vi "Coffee_Main.vi"() -> ()   [LabVIEW 2020]
doc: "This VI performs the application of coffee machine controller where user can choose the beverage."
uses:
  Controls/QueueOperations.ctl
  Controls/DataCluster.ctl
  <vilib>/Utility/config.llb/Read Key (Boolean).vi
  <vilib>/Utility/config.llb/Read Key (I32).vi
  <vilib>/Utility/config.llb/Read Key (Double).vi
  <vilib>/Utility/config.llb/NI_LVConfig.lvlib
panel:
  in  "Power":bool
  out "error out":errorcluster
  in  "error in (no error)":errorcluster
  in  "Dispenser":dbl(slide) scale=0.0..60.0
  in  "Chamber":dbl(slide) scale=0.0..60.0
  out "Milk level":dbl(slide) scale=0.0..100.0
  out "Water Level":dbl(slide) scale=0.0..100.0
  out "Bean Level":dbl(slide) scale=0.0..100.0
  out "Total Cups":i32
  out "Elapsed Time":dbl
  out "Dispensing":bool
  out "Brewing":bool
  out "Grinding":bool
  out "Purging":bool
  out "Heating":bool
  out "Low Milk":bool
  out "Low Bean":bool
  out "Low Water":bool
  in  "1 Carale":bool
  in  "1 Cup":bool
  in  "Knob":i32(knob) scale=0.0..2.0
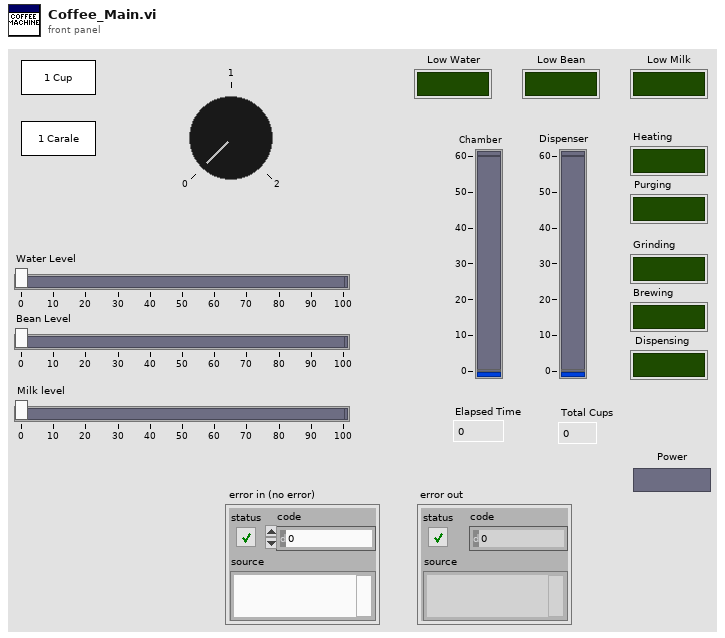
[diagram p1: front panel]
types:
  T1 = typedef "DataCluster.ctl" = cluster{"Brewing":bool, "Grinding":bool, "Purging":bool, "Dispensing":bool, "Heating":bool, "Low Milk":bool, "Low Bean":bool, "Low Water":bool, "Path":path, "Power On?":bool, "Proper Shutdown?":bool, "Total Cups":i32, "Start Time":dbl, "Elapsed Time":dbl, "Bean Level":dbl, "Milk Level":dbl, "Water Level":dbl, "HeatTime":dbl, "Beverage Type":string, "Steps":string[], "Time Sequence":dbl[], "Index":i32}
  T2 = typedef "QueueOperations.ctl" = enum16{"Create", "Enqueue", "Enqueue N", "Enstack", "Dequeue", "Flush", "Release"}
  T3 = typedef "NI_LVConfig.lvlib/Config Data RefNum.ctl" = refnum<k1>
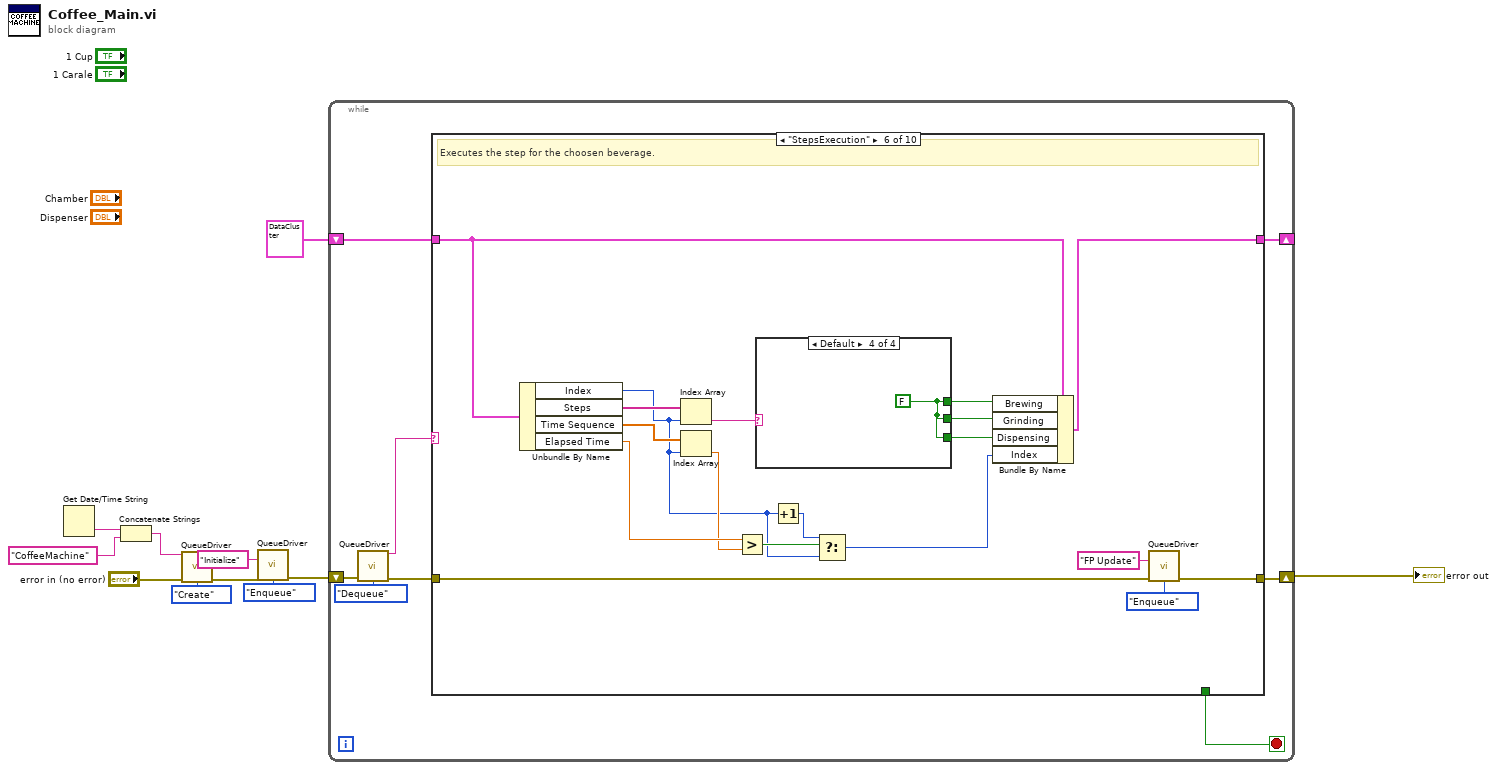
[diagram p0: block diagram]
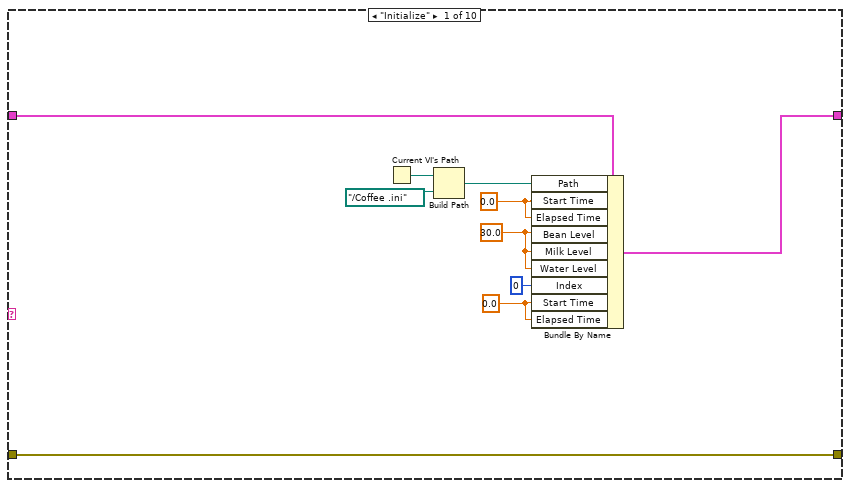
[diagram p2: hidden frame]
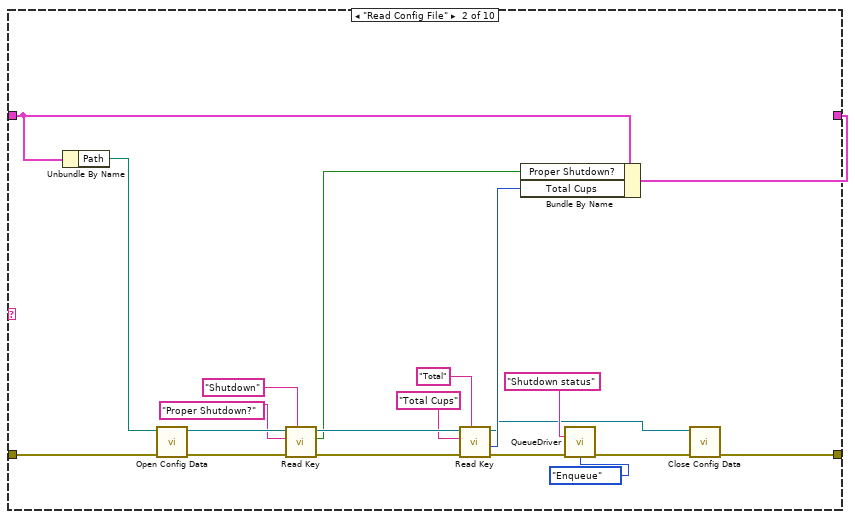
[diagram p3: hidden frame]
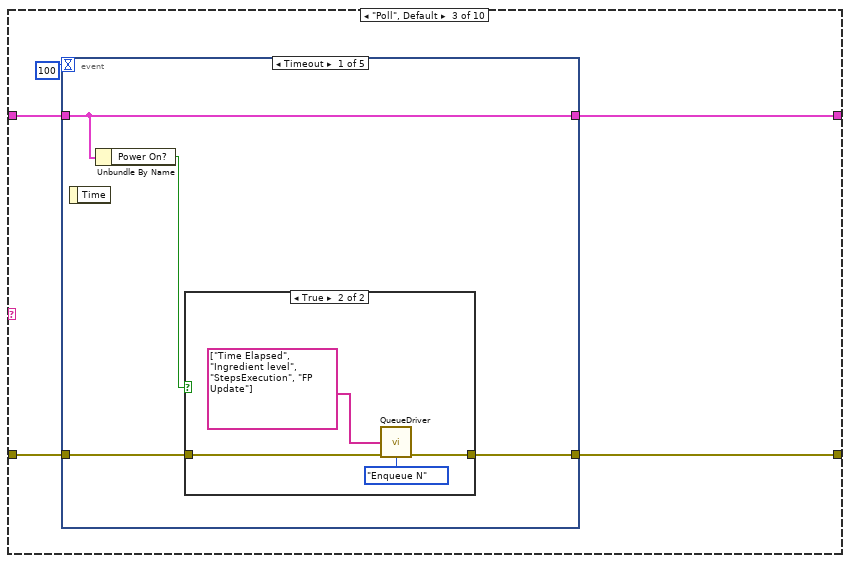
[diagram p4: hidden frame]
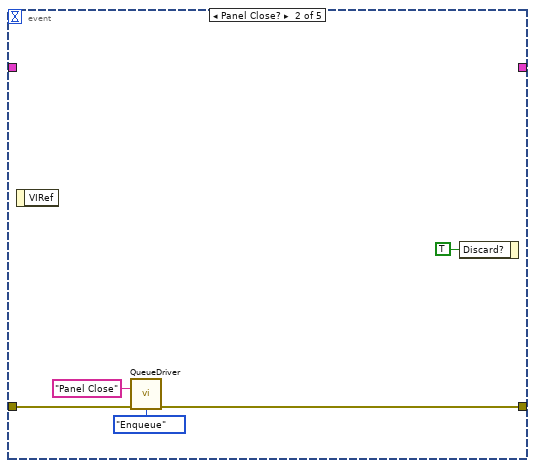
[diagram p6: hidden frame]
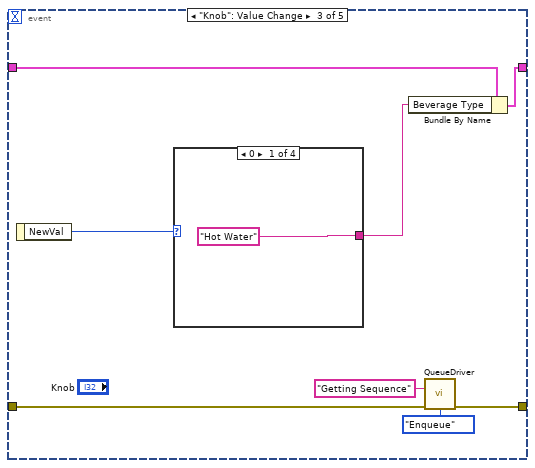
[diagram p7: hidden frame]
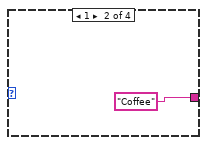
[diagram p8: hidden frame]
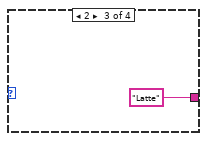
[diagram p9: hidden frame]
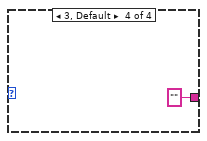
[diagram p10: hidden frame]
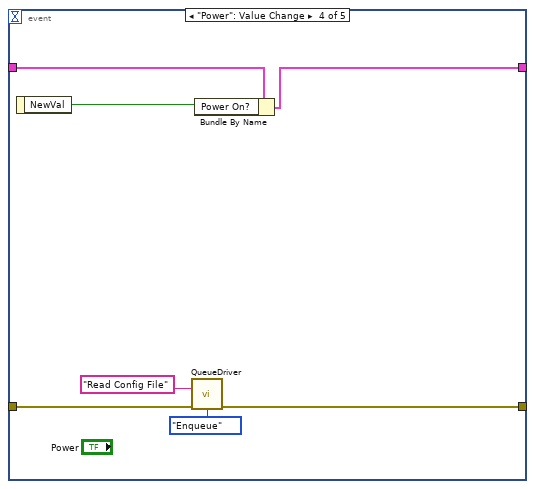
[diagram p11: hidden frame]
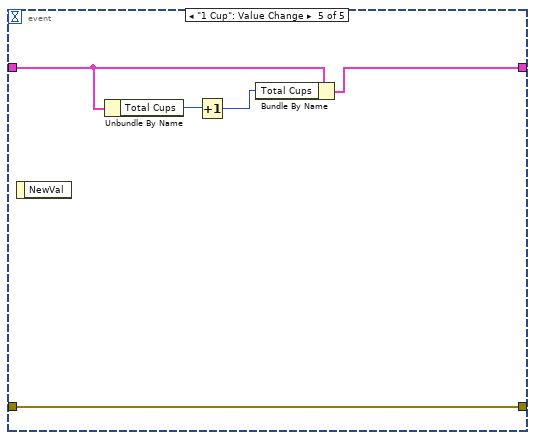
[diagram p12: hidden frame]
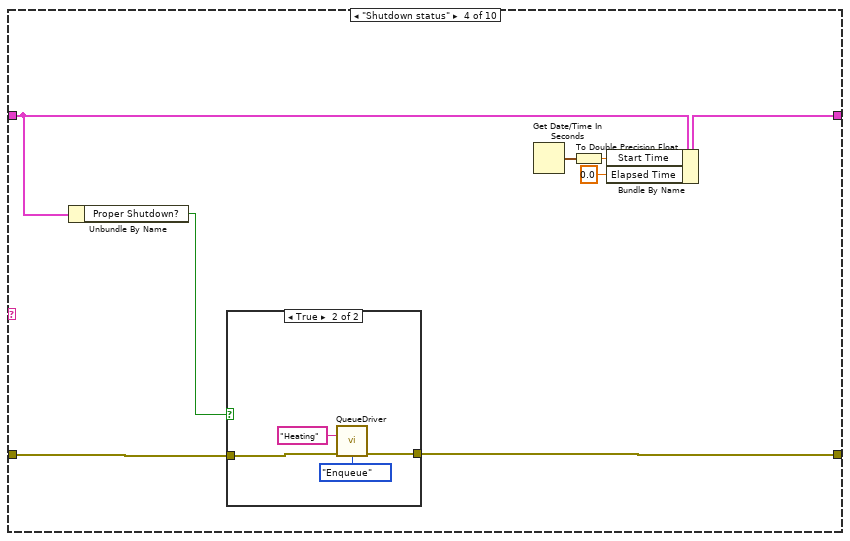
[diagram p13: hidden frame]
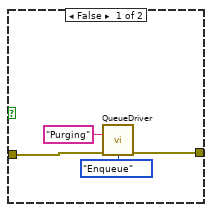
[diagram p14: hidden frame]
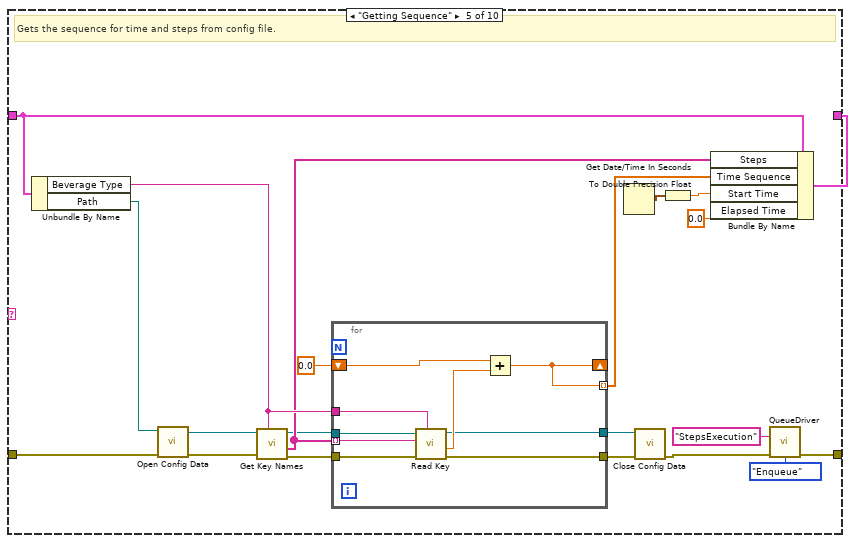
[diagram p15: hidden frame]
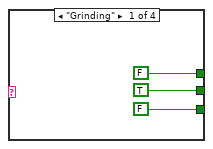
[diagram p16: hidden frame]
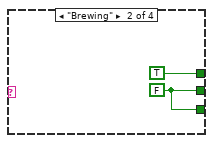
[diagram p17: hidden frame]
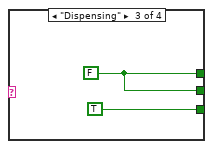
[diagram p18: hidden frame]
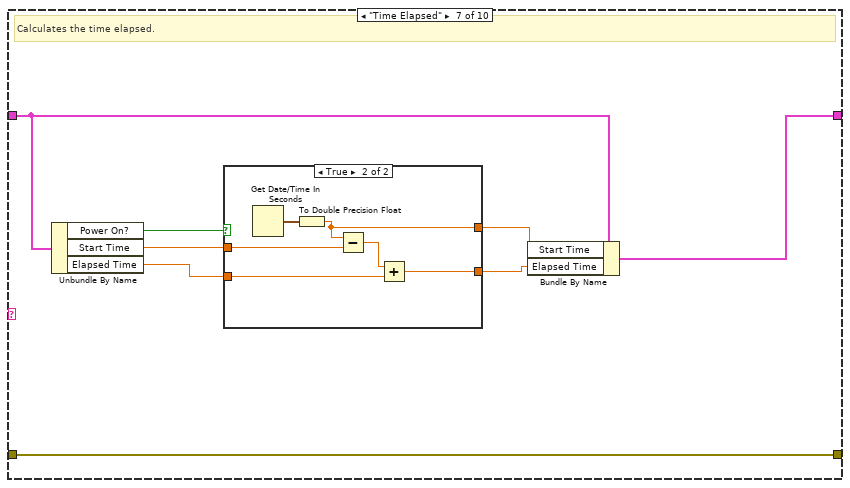
[diagram p19: hidden frame]
diagram:
  n1 = Get Date/Time String() -> (time string=w9:string)  [unwired: 3 in, 1 out]
  n2 = Concatenate Strings(w9, "CoffeeMachine" ("Queue Name")) -> (w10:string)
  n3 = call "QueueDriver.vi"("Queue Name"=w10, "error in (no error)"="error in (no error)", "Operation"=QueueOperations."Create") -> ("error out"=w6:errorcluster)  [unwired: 11 in, 1 out]
  n4 = call "QueueDriver.vi"("State"="Initialize", "error in (no error)"=w6, "Operation"=QueueOperations."Enqueue") -> ("error out"=w4:errorcluster)  [unwired: 11 in, 1 out]
  n5 = while {
    shift-right: [w14] -> _
    shift-left: T1 {"Brewing"=FALSE, "Grinding"=FALSE, "Purging"=FALSE, "Dispensing"=FALSE, "Heating"=FALSE, "Low Milk"=FALSE, "Low Bean"=FALSE, "Low Water"=FALSE, "Path"=path "", "Power On?"=FALSE, "Proper Shutdown?"=FALSE, "Total Cups"=0, "Start Time"=0.0, "Elapsed Time"=0.0, "Bean Level"=0.0, "Milk Level"=0.0, "Water Level"=0.0, "HeatTime"=0.0, "Beverage Type"="", "Steps"=[], "Time Sequence"=[], "Index"=0} -> [w15]
    shift-right: [w13] -> w2
    shift-left: w4 -> [w19]
    stop <- w12 stop-if-true
    n6 = call "QueueDriver.vi"("error in (no error)"=w19, "Operation"=QueueOperations."Dequeue") -> ("Dequeued Element"=w17:string, "error out"=w16:errorcluster)  [unwired: 12 in]
    n7 = case shown="\"StepsExecution\"" w17 {
      tunnel: w16 -> [w24 w48 w51 w100 w129 w142 w166 w181 w196 w211]
      tunnel: w15 -> [w27 w39 w53 w97 w124 w153 w170 w186 w197 w212]
      tunnel: [w26 w33 w52 w96 w119 w152 w167 w182 w197 w212] -> w14
      tunnel: [w24 w31 w50 w99 w117 w141 w166 w181 w192 w211] -> w13
      tunnel: [_ _ _ _ _ _ _ _ TRUE _] -> w12
      frame "Initialize" {
        w20 = 0.0 ("Start Time")
        w22 = 30.0 ("Bean Level")
        w23 = 0.0 ("Start Time")
        n8 = Current VI's Path() -> (path=w29:path)
        n9 = Build Path(base path=w29, name or relative path=path "../Coffee .ini") -> (appended path=w25:path)
        n10 = Bundle By Name(cluster=w27, "Path"=w25, "Start Time"=w23, "Elapsed Time"=w23, "Bean Level"=w22, "Milk Level"=w22, "Water Level"=w22, "Index"=0, "Start Time"=w20, "Elapsed Time"=w20) -> (w26:T1)
      }
      frame "Read Config File" {
        n11 = Unbundle By Name(w39) -> ("Path"=w49:path)
        n12 = call <vilib>:"Open Config Data.vi"("error in (no error)"=w48, "configuration file path"=w49) -> ("error out"=w43:errorcluster, "refnum"=w47:T3)  [unwired: 7 in, 1 out]
        n13 = call-poly <vilib>:"Read Key.vi"("section"="Shutdown", "error in (no error)"=w43, "key"="Proper Shutdown?", "refnum"=w47) -> ("error out"=w42:errorcluster, "found?"=w38:bool, "refnum out"=w45:T3)  [unwired: 4 in, 1 out]
        n14 = call-poly <vilib>:"Read Key.vi"("section"="Total", "error in (no error)"=w42, "key"="Total Cups", "refnum"=w45) -> ("error out"=w36:errorcluster, "value"=w37:i32, "refnum out"=w30:T3)  [unwired: 4 in, 1 out]
        n15 = Bundle By Name(cluster=w39, "Proper Shutdown?"=w38, "Total Cups"=w37) -> (w33:T1)
        n16 = call "QueueDriver.vi"("State"="Shutdown status", "error in (no error)"=w36, "Operation"=QueueOperations."Enqueue") -> ("error out"=w32:errorcluster)  [unwired: 11 in, 1 out]
        n17 = call <vilib>:"Close Config Data.vi"("error in (no error)"=w32, "refnum"=w30) -> ("error out"=w31:errorcluster)  [unwired: 8 in, 1 out]
      }
      frame "Poll", Default {
        n18 = event shown="[0] Timeout" {
          selector: _ -> [_ _ _ _ _]
          dyn-events: _ -> [_ _ _ _ _]
          timeout: 100 -> [_ _ _ _ _]
          tunnel: w53 -> [w56 _ w75 w87 w91]
          tunnel: [w56 _ w74 w85 w92] -> w52
          tunnel: w51 -> [w58 w67 w72 w84 w88]
          tunnel: [w57 w66 w71 w81 w88] -> w50
          event Timeout {
            n19 = event-data() -> ()  [unwired: 1 in, 1 out]
            n20 = Unbundle By Name(w56) -> ("Power On?"=w55:bool)
            n21 = case shown="True" w55 {
              tunnel: w58 -> [w59 w63]
              tunnel: [w59 w62] -> w57
              frame False {
              }
              frame True {
                n22 = call "QueueDriver.vi"("State  s[]"=string[] ["Time Elapsed", "Ingredient level", "StepsExecution", "FP Update"], "error in (no error)"=w63, "Operation"=QueueOperations."Enqueue N") -> ("error out"=w62:errorcluster)  [unwired: 11 in, 1 out]
              }
            }
          }
          event Panel Close? {
            n23 = event-data() -> ()  [unwired: 1 in, 1 out]
            n24 = call "QueueDriver.vi"("State"="Panel Close", "error in (no error)"=w67, "Operation"=QueueOperations."Enqueue") -> ("error out"=w66:errorcluster)  [unwired: 11 in, 1 out]
            n25 = event-data("Discard?"=TRUE) -> ()  [unwired: 1 in, 1 out]
          }
          event "Knob": Value Change {
            n26 = event-data() -> ("NewVal"=w76:i32)  [unwired: 1 in]
            n27 = case shown="0" w76 {
              tunnel: ["Hot Water" "Coffee" "Latte" ""] -> w73
              frame 0 {
              }
              frame 1 {
              }
              frame 2 {
              }
              frame 3, Default {
              }
            }
            n28 = Bundle By Name(cluster=w75, "Beverage Type"=w73) -> (w74:T1)
            n29 = call "QueueDriver.vi"("State"="Getting Sequence", "error in (no error)"=w72, "Operation"=QueueOperations."Enqueue") -> ("error out"=w71:errorcluster)  [unwired: 11 in, 1 out]
          }
          event "Power": Value Change {
            n30 = event-data() -> ("NewVal"=w86:bool)  [unwired: 1 in]
            n31 = call "QueueDriver.vi"("State"="Read Config File", "error in (no error)"=w84, "Operation"=QueueOperations."Enqueue") -> ("error out"=w81:errorcluster)  [unwired: 11 in, 1 out]
            n32 = Bundle By Name(cluster=w87, "Power On?"=w86) -> (w85:T1)
          }
          event "1 Cup": Value Change {
            n33 = event-data() -> ()  [unwired: 1 in, 1 out]
            n34 = Unbundle By Name(w91) -> ("Total Cups"=w90:i32)
            n35 = Increment(x=w90) -> (x+1=w89:i32)
            n36 = Bundle By Name(cluster=w91, "Total Cups"=w89) -> (w92:T1)
          }
        }
      }
      frame "Shutdown status" {
        n37 = Unbundle By Name(w97) -> ("Proper Shutdown?"=w98:bool)
        n38 = case shown="True" w98 {
          tunnel: w100 -> [w104 w107]
          tunnel: [w103 w106] -> w99
          frame False {
            n39 = call "QueueDriver.vi"("State"="Purging", "error in (no error)"=w104, "Operation"=QueueOperations."Enqueue") -> ("error out"=w103:errorcluster)  [unwired: 11 in, 1 out]
          }
          frame True {
            n40 = call "QueueDriver.vi"("State"="Heating", "error in (no error)"=w107, "Operation"=QueueOperations."Enqueue") -> ("error out"=w106:errorcluster)  [unwired: 11 in, 1 out]
          }
        }
        n41 = Get Date/Time In Seconds() -> (seconds since 1Jan1904=w95:timestamp)
        n42 = To Double Precision Float(number=w95) -> (double precision float=w94:dbl)
        n43 = Bundle By Name(cluster=w97, "Start Time"=w94, "Elapsed Time"=0.0) -> (w96:T1)
      }
      frame "Getting Sequence" {
        # "Gets the sequence for time and steps from config file."
        n44 = Unbundle By Name(w124) -> ("Beverage Type"=w122:string, "Path"=w128:path)
        n45 = call <vilib>:"Open Config Data.vi"("error in (no error)"=w129, "configuration file path"=w128) -> ("error out"=w127:errorcluster, "refnum"=w126:T3)  [unwired: 7 in, 1 out]
        n46 = call <vilib>:"Get Key Names.vi"("section"=w122, "error in (no error)"=w127, "refnum"=w126) -> ("error out"=w123:errorcluster, "key names"=w120:string[], "refnum out"=w118:T3)  [unwired: 5 in, 1 out]
        n47 = for {
          shift-right: [w133] -> _
          shift-left: 0.0 -> [w135]
          tunnel: w123 -> [w138]
          tunnel: w120 -> [w137] mode=indexing
          tunnel: w122 -> [w136]
          tunnel: [w133] -> w121 mode=indexing
          tunnel: [w132] -> w111
          tunnel: w118 -> [w131]
          tunnel: [w130] -> w109
          n48 = call-poly <vilib>:"Read Key.vi"("section"=w136, "error in (no error)"=w138, "key"=w137, "refnum"=w131) -> ("error out"=w132:errorcluster, "value"=w134:dbl, "refnum out"=w130:T3)  [unwired: 4 in, 1 out]
          n49 = Add(x=w135, y=w134) -> (x+y=w133:dbl)
        }
        n50 = Get Date/Time In Seconds() -> (seconds since 1Jan1904=w113:timestamp)
        n51 = call <vilib>:"Close Config Data.vi"("error in (no error)"=w111, "refnum"=w109) -> ("error out"=w110:errorcluster)  [unwired: 8 in, 1 out]
        n52 = To Double Precision Float(number=w113) -> (double precision float=w114:dbl)
        n53 = Bundle By Name(cluster=w124, "Steps"=w120, "Time Sequence"=w121, "Start Time"=w114, "Elapsed Time"=0.0) -> (w119:T1)
        n54 = call "QueueDriver.vi"("State"="StepsExecution", "error in (no error)"=w110, "Operation"=QueueOperations."Enqueue") -> ("error out"=w117:errorcluster)  [unwired: 11 in, 1 out]
      }
      frame "StepsExecution" {
        # "Executes the step for the choosen beverage."
        n55 = Unbundle By Name(w153) -> ("Index"=w144:i32, "Steps"=w156:string[], "Time Sequence"=w155:dbl[], "Elapsed Time"=w148:dbl)
        n56 = Index Array(array=w156, index=w144) -> (element=w154:string)
        n57 = Index Array(array=w155, index=w144) -> (element=w147:dbl)
        n58 = Greater?(x=w148, y=w147) -> (0:w146:bool)
        n59 = case shown="Default" w154 {
          tunnel: [TRUE w161 w163 w164] -> w151
          tunnel: [FALSE w161 TRUE w164] -> w150
          tunnel: [FALSE TRUE w163 w164] -> w149
          frame "Grinding" {
          }
          frame "Brewing" {
            w161 = FALSE
          }
          frame "Dispensing" {
            w163 = FALSE
          }
          frame Default {
            w164 = FALSE
          }
        }
        n60 = Increment(x=w144) -> (x+1=w145:i32)
        n61 = Select(t=w145, s=w146, f=w144) -> (s? t:f=w143:i32)
        n62 = Bundle By Name(cluster=w153, "Brewing"=w149, "Grinding"=w151, "Dispensing"=w150, "Index"=w143) -> (w152:T1)
        n63 = call "QueueDriver.vi"("State"="FP Update", "error in (no error)"=w142, "Operation"=QueueOperations."Enqueue") -> ("error out"=w141:errorcluster)  [unwired: 11 in, 1 out]
      }
      frame "Time Elapsed" {
        # "Calculates the time elapsed."
        n64 = Unbundle By Name(w170) -> ("Power On?"=w172:bool, "Start Time"=w171:dbl, "Elapsed Time"=w165:dbl)
        n65 = case shown="True" w172 {
          tunnel: w171 -> [w174 w179]
          tunnel: w165 -> [w173 w177]
          tunnel: [w174 w176] -> w169
          tunnel: [w173 w175] -> w168
          frame False {
          }
          frame True {
            n66 = Get Date/Time In Seconds() -> (seconds since 1Jan1904=w180:timestamp)
            n67 = To Double Precision Float(number=w180) -> (double precision float=w176:dbl)
            n68 = Subtract(x=w176, y=w179) -> (x-y=w178:dbl)
            n69 = Add(x=w178, y=w177) -> (x+y=w175:dbl)
          }
        }
        n70 = Bundle By Name(cluster=w170, "Start Time"=w169, "Elapsed Time"=w168) -> (w167:T1)
      }
      frame "Ingredient level" {
        w187 = 30.0 ("y")
        # "Checks the ingredient level."
        n71 = Unbundle By Name(w186) -> ("Milk Level"=w190:dbl, "Bean Level"=w189:dbl, "Water Level"=w188:dbl)
        n72 = Less?(x=w190, y=w187) -> (x < y?=w185:bool)
        n73 = Less?(x=w189, y=w187) -> (x < y?=w184:bool)
        n74 = Less?(x=w188, y=w187) -> (x < y?=w183:bool)
        n75 = Bundle By Name(cluster=w186, "Low Milk"=w185, "Low Bean"=w184, "Low Water"=w183) -> (w182:T1)
      }
      frame "Panel Close" {
        n76 = call "QueueDriver.vi"("error in (no error)"=w196, "Operation"=QueueOperations."Flush") -> ("error out"=w193:errorcluster)  [unwired: 12 in, 1 out]
        n77 = call "QueueDriver.vi"("error in (no error)"=w193, "Operation"=QueueOperations."Release") -> ("error out"=w192:errorcluster)  [unwired: 12 in, 1 out]
      }
      frame "FP Update" {
        n78 = Unbundle By Name(w212) -> ("Elapsed Time"=→"Elapsed Time":dbl, "Heating"=→"Heating":bool, "Bean Level"=→"Bean Level":dbl, "Milk Level"=→"Water Level":dbl, "Water Level"=→"Milk level":dbl, "Low Milk"=→"Low Milk":bool, "Low Bean"=→"Low Bean":bool, "Low Water"=→"Low Water":bool, "Total Cups"=→"Total Cups":i32, "Grinding"=→"Grinding":bool, "Brewing"=→"Brewing":bool, "Dispensing"=→"Dispensing":bool, "Purging"=→"Purging":bool)
      }
    }
  }
  "error out" <- w2
